vi "niFpga wdp fft pfft 4.vi"(6 "enable":bool, 11 "data in":T1(array[cluster])=[{"data re"=0.0, "data im"=0.0}, {"data re"=0.0, "data im"=0.0}, {"data re"=0.0, "data im"=0.0}, {"data re"=0.0, "data im"=0.0}]) -> (3 "data out":T2(array[cluster]))   [LabVIEW 2017]
types:
  T1 = cluster{"data re":fxp<+/-,8,1>, "data im":fxp<+/-,8,1>}[]
  T2 = cluster{"data re":fxp<+/-,8,1>, "data re":fxp<+/-,8,1>}[]
  T3 = cluster{"data re":fxp<+/-,8,1>, "data im":fxp<+/-,8,1>}
  T4 = cluster{"data re":fxp<+/-,8,1>, "data re":fxp<+/-,8,1>}
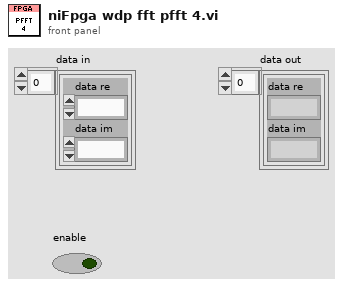
[diagram p1: front panel]
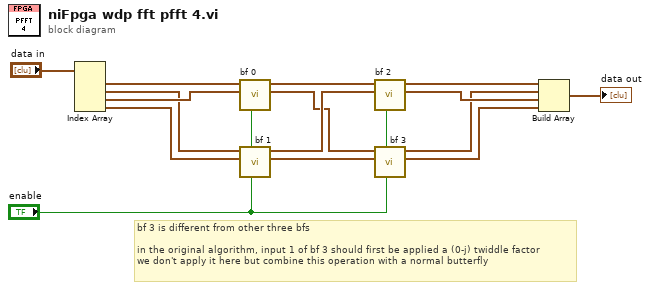
[diagram p0: block diagram]
diagram:
  # "bf 3 is different from other three bfs\n\nin the original algorithm, input 1 of bf 3 should first be applied a (0-j) twiddle factor\nwe don't apply it here but combine this operation with a normal butterfly"
  n1 = Index Array(array="data in") -> (element #1=w8:T3, element #2=w9:T3, element #3=w10:T3, element #4=w11:T3)  [unwired: 4 in]
  n2 = call "bf 0"("enable"="enable", "data in 1"=w10, "data in 0"=w8) -> ("data out 1"=w2:T4, "data out 0"=w5:T4)  [unwired: 7 in]
  n3 = call "bf 1"("enable"="enable", "data in 1"=w11, "data in 0"=w9) -> ("data out 1"=w3:T4, "data out 0"=w4:T4)  [unwired: 7 in]
  n4 = call "bf 2"("enable"="enable", "data in 1"=w4, "data in 0"=w5) -> ("data out 1"=w14:T4, "data out 0"=w12:T4)  [unwired: 7 in]
  n5 = call "bf 3"("enable"="enable", "data in 1"=w3, "data in 0"=w2) -> ("data out 1"=w15:T4, "data out 0"=w13:T4)  [unwired: 7 in]
  n6 = Build Array(w12, w13, w14, w15) -> (→"data out":T2)
